vi "globals.vi"() -> ()   [LabVIEW 2015]
panel:
  out "camera-right":T1(plugin-control)
  out "camera-left":T1(plugin-control)
  out "Exposure time":dbl
  in  "Stop Button":bool
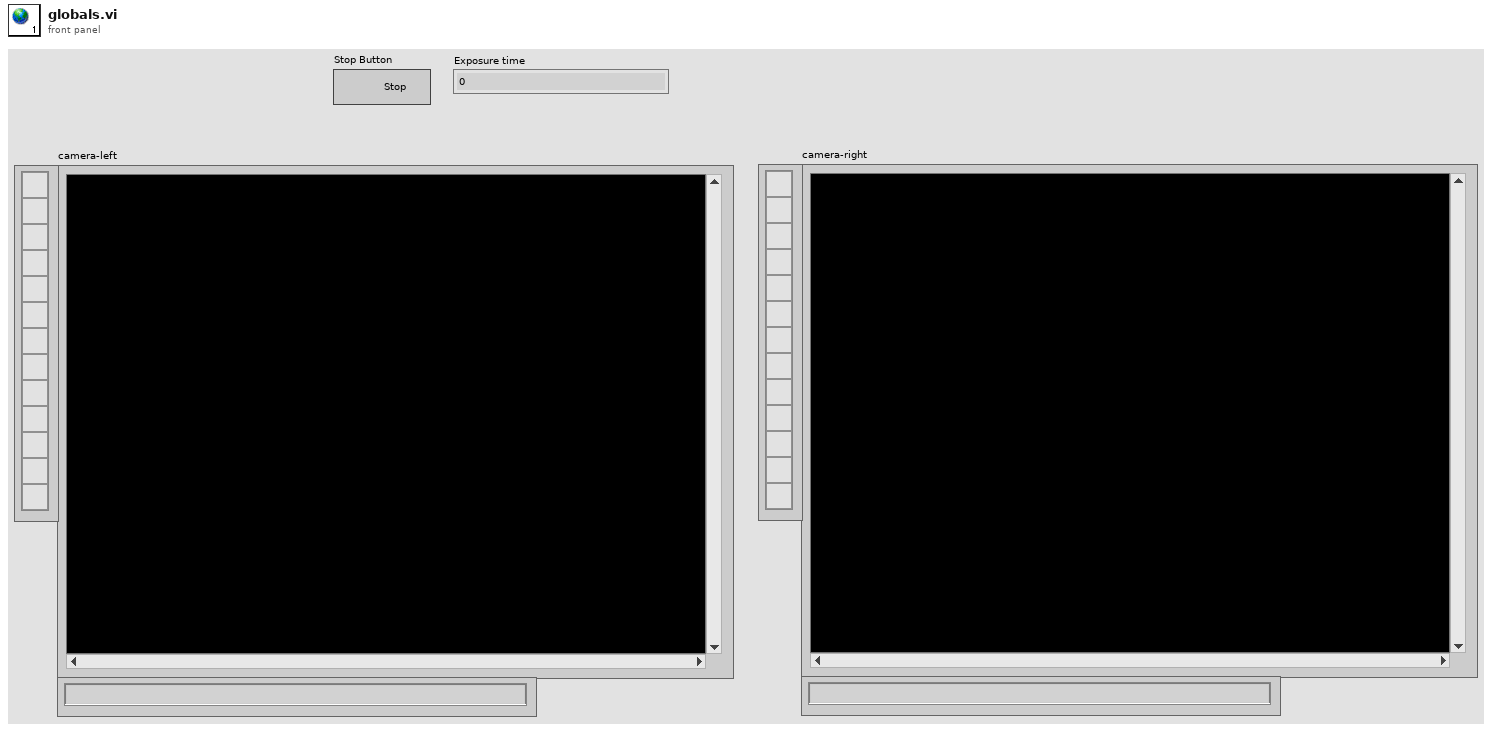
[diagram p1: front panel]
types:
  T1 = typedef "IMAQ Image.ctl" = refnum<image>
diagram:
